vi "Loop Speed.vi"(1 "milliseconds to wait":u32=10) -> (0 "Swerve-Loop Speed":u32)   [LabVIEW 2015]
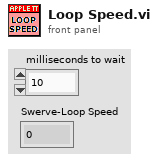
[diagram p1: front panel]
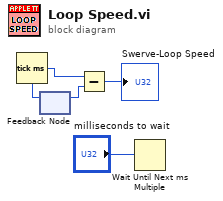
[diagram p0: block diagram]
diagram:
  n1 = Tick Count (ms)() -> (millisecond timer value=w3:u32)
  n2 = feedback #1() -> (w4:u32)  [unwired: 1 in]
  n3 = feedback-in #1(w3) -> ()
  n4 = Subtract(x=w3, y=w4) -> (x-y=→"Swerve-Loop Speed":u32)
  n5 = Wait Until Next ms Multiple(millisecond multiple="milliseconds to wait") -> ()  [unwired: 1 out]
